vi "Smart Scan from String.vi"(0 "initial string":string, 1 "Syntax Format":T1={"Syntax"="", "Variable#"=enum."One"}, 11 "error in":errorcluster) -> (4 "resulting string":string, 6 "Variables":string[](array[string]), 15 "error out":errorcluster)   [LabVIEW 2016]
uses:
  Syntax Format.ctl
  Variable#.ctl
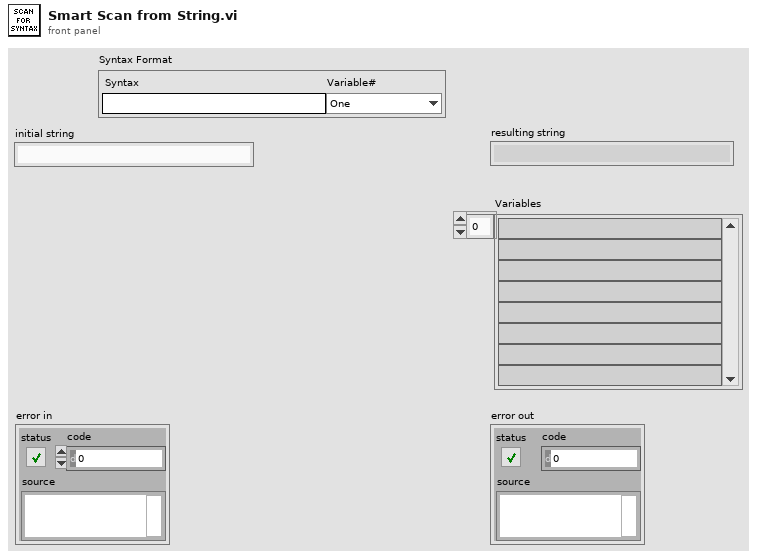
[diagram p1: front panel]
types:
  T1 = typedef "Syntax Format.ctl" = cluster{"Syntax":string, "Variable#":T2}
  T2 = typedef "Variable#.ctl" = enum16{"Zero", "One", "Two", "Three", "Four", "Five"}
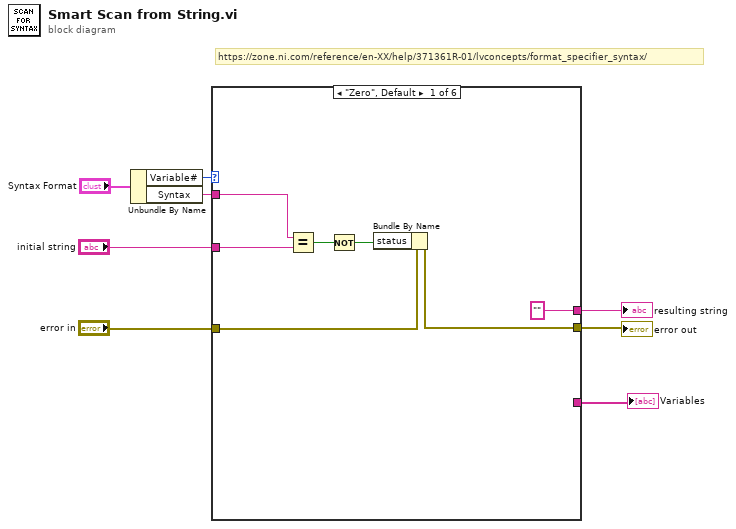
[diagram p0: block diagram]
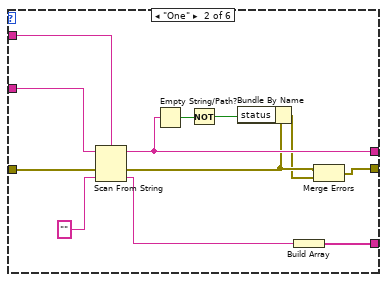
[diagram p2: hidden frame]
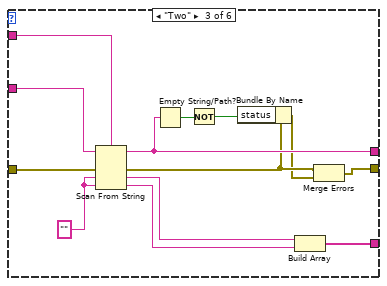
[diagram p3: hidden frame]
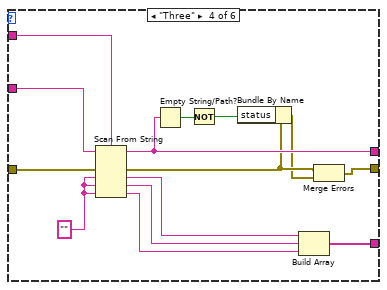
[diagram p4: hidden frame]
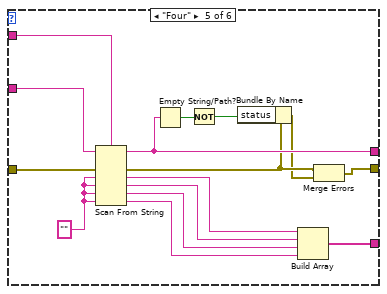
[diagram p5: hidden frame]
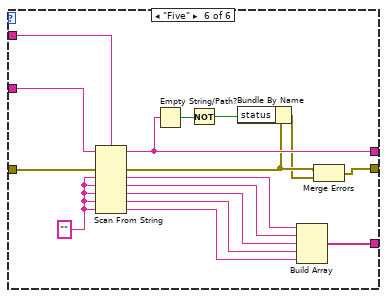
[diagram p6: hidden frame]
diagram:
  # "https://zone.ni.com/reference/en-XX/help/371361R-01/lvconcepts/format_specifier_syntax/"
  n1 = Unbundle By Name("Syntax Format") -> ("Variable#"=w3:T2, "Syntax"=w4:string)
  n2 = case shown="\"Zero\", Default" w3 {
    tunnel: "initial string" -> [w14 w27 w40 w54 w69 w85]
    tunnel: "error in" -> [w12 w25 w39 w53 w68 w84]
    tunnel: ["" w24 w38 w52 w67 w83] -> w6
    tunnel: [w11 w18 w32 w46 w61 w77] -> w2
    tunnel: w4 -> [w15 w21 w35 w49 w64 w80]
    tunnel: [_ w16 w28 w41 w55 w70] -> w1
    frame "Zero", Default {
      n3 = Equal?(x=w15, y=w14) -> (x = y?=w10:bool)
      n4 = Not(x=w10) -> (.not. x?=w9:bool)
      n5 = Bundle By Name(cluster=w12, "status"=w9) -> (w11:errorcluster)
    }
    frame "One" {
      n6 = Scan From String(format string=w21, input string=w27, error in=w25, default 1="") -> (remaining string=w24:string, error out=w20:errorcluster, output 1=w17:string)  [unwired: 1 in, 1 out]
      n7 = Empty String/Path?(string/path=w24) -> (empty?=w23:bool)
      n8 = Not(x=w23) -> (.not. x?=w22:bool)
      n9 = Bundle By Name(cluster=w20, "status"=w22) -> (w19:errorcluster)
      n10 = Build Array(w17) -> (w16:string[])
      n11 = Merge Errors(w20, w19) -> (w18:errorcluster)
    }
    frame "Two" {
      w31 = ""
      n12 = Scan From String(format string=w35, input string=w40, error in=w39, default 1=w31, default 2=w31) -> (remaining string=w38:string, error out=w34:errorcluster, output 1=w30:string, output 2=w29:string)  [unwired: 1 in, 1 out]
      n13 = Empty String/Path?(string/path=w38) -> (empty?=w37:bool)
      n14 = Not(x=w37) -> (.not. x?=w36:bool)
      n15 = Bundle By Name(cluster=w34, "status"=w36) -> (w33:errorcluster)
      n16 = Build Array(w30, w29) -> (w28:string[])
      n17 = Merge Errors(w34, w33) -> (w32:errorcluster)
    }
    frame "Three" {
      w45 = ""
      n18 = Scan From String(format string=w49, input string=w54, error in=w53, default 1=w45, default 2=w45, default 3=w45) -> (remaining string=w52:string, error out=w48:errorcluster, output 1=w44:string, output 2=w43:string, output 3=w42:string)  [unwired: 1 in, 1 out]
      n19 = Empty String/Path?(string/path=w52) -> (empty?=w51:bool)
      n20 = Not(x=w51) -> (.not. x?=w50:bool)
      n21 = Bundle By Name(cluster=w48, "status"=w50) -> (w47:errorcluster)
      n22 = Build Array(w44, w43, w42) -> (w41:string[])
      n23 = Merge Errors(w48, w47) -> (w46:errorcluster)
    }
    frame "Four" {
      w60 = ""
      n24 = Scan From String(format string=w64, input string=w69, error in=w68, default 1=w60, default 2=w60, default 3=w60, default 4=w60) -> (remaining string=w67:string, error out=w63:errorcluster, output 1=w59:string, output 2=w58:string, output 3=w57:string, output 4=w56:string)  [unwired: 1 in, 1 out]
      n25 = Empty String/Path?(string/path=w67) -> (empty?=w66:bool)
      n26 = Not(x=w66) -> (.not. x?=w65:bool)
      n27 = Bundle By Name(cluster=w63, "status"=w65) -> (w62:errorcluster)
      n28 = Build Array(w59, w58, w57, w56) -> (w55:string[])
      n29 = Merge Errors(w63, w62) -> (w61:errorcluster)
    }
    frame "Five" {
      w76 = ""
      n30 = Scan From String(format string=w80, input string=w85, error in=w84, default 1=w76, default 2=w76, default 3=w76, default 4=w76, default 5=w76) -> (remaining string=w83:string, error out=w79:errorcluster, output 1=w75:string, output 2=w74:string, output 3=w73:string, output 4=w72:string, output 5=w71:string)  [unwired: 1 in, 1 out]
      n31 = Empty String/Path?(string/path=w83) -> (empty?=w82:bool)
      n32 = Not(x=w82) -> (.not. x?=w81:bool)
      n33 = Bundle By Name(cluster=w79, "status"=w81) -> (w78:errorcluster)
      n34 = Build Array(w75, w74, w73, w72, w71) -> (w70:string[])
      n35 = Merge Errors(w79, w78) -> (w77:errorcluster)
    }
  }
  "resulting string" <- w6
  "error out" <- w2
  "Variables" <- w1
